vi "FirePneumaticQueue.vi"(8 "error in (no error)":errorcluster, 10 "Variant":variant) -> (0 "error out":errorcluster)   [LabVIEW 2012]
uses:
  RefnameEnum.ctl
  <vilib>/Rock Robotics/WPI/Solenoid/WPI_SolenoidValue.ctl
  <vilib>/Rock Robotics/WPI/Solenoid/WPI_SolenoidSetEnum.vi
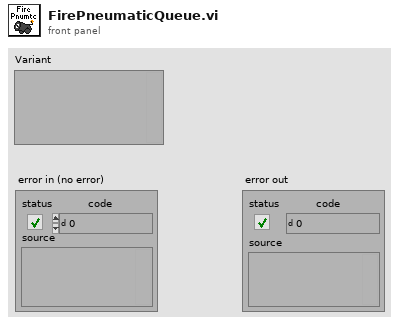
[diagram p1: front panel]
types:
  T1 = typedef "WPI_SolenoidValue.ctl" = enum16{"Off", "On", "Forward", "Reverse"}
  T2 = typedef "RefnameEnum.ctl" = enum16{"FireLauncher", "Climber", "Shield", "TankDrive", "DriveEncoderL", "DriveEncoderR", "LauncherMotorRPM", "LauncherEncoderAnalog", "LauncherEncoderRPM", "ShooterLS", "DriveAlignLSLeft", "DriveAlignLSRight", "ClimbingLS", "LauncherEncoderAngle", "LauncherMotorAngle", "Gamepad1", "Gamepad2", "Compressor", "ClimbWeightSol3", "ClimbWeightSol4"}
  T3 = typedef "WPI_SolenoidDevRef.ctl" = cluster{"DevStatus":errorcluster, "Solenoid Module":T4, "Forward Solenoid Channel":T5, "Reverse Solenoid Channel":T5}
  T4 = typedef "FPGA_TypedefSolenoidModule.ctl" = enum16{"Solenoid Module 1", "Solenoid Module 2"}
  T5 = typedef "WPI_SolenoidChannel.ctl" = enum8{"Solenoid 1", "Solenoid 2", "Solenoid 3", "Solenoid 4", "Solenoid 5", "Solenoid 6", "Solenoid 7", "Solenoid 8", "Invalid"}
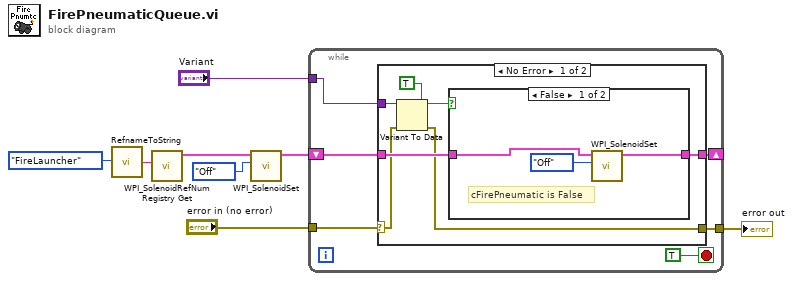
[diagram p0: block diagram]
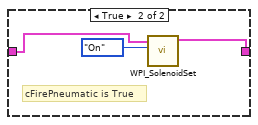
[diagram p2: hidden frame]
diagram:
  n1 = call "RefnameToString.vi"("Enum"=RefnameEnum."FireLauncher") -> ("Refname"=w6:string)
  n2 = call <vilib>:"WPI_SolenoidRefNum Registry Get.vi"("refnum name"=w6) -> ("SolenoidDevRef"=w8:T3)  [unwired: 9 in, 1 out]
  n3 = call-poly <vilib>:"WPI_SolenoidSet.vi"("Value"=WPI_SolenoidValue."Off", "SolenoidDevRef"=w8) -> ("SolenoidDevRef"=w5:T3)  [unwired: 1 in, 8 out]
  n4 = while {
    shift-right: [w13] -> _
    shift-left: w5 -> [w14]
    tunnel: "Variant" -> [w10]
    tunnel: "error in (no error)" -> [w11]
    tunnel: [w9] -> w1
    stop <- TRUE stop-if-true
    n5 = case shown="No Error" w11 {
      selector: w11 -> [w17 w28]
      tunnel: w14 -> [w19 w29]
      tunnel: [w18 w29] -> w13
      tunnel: w10 -> [w16 _]
      tunnel: [w15 w28] -> w9
      frame No Error {
        n6 = Variant To Data(error in=w17, type=TRUE, Variant=w16) -> (data=w20:bool, error out=w15:errorcluster)
        n7 = case shown="False" w20 {
          tunnel: w19 -> [w23 w26]
          tunnel: [w22 w25] -> w18
          frame False {
            # "cFirePneumatic is False"
            n8 = call-poly <vilib>:"WPI_SolenoidSet.vi"("Value"=WPI_SolenoidValue."Off", "SolenoidDevRef"=w23) -> ("SolenoidDevRef"=w22:T3)  [unwired: 1 in, 8 out]
          }
          frame True {
            # "cFirePneumatic is True"
            n9 = call-poly <vilib>:"WPI_SolenoidSet.vi"("Value"=WPI_SolenoidValue."On", "SolenoidDevRef"=w26) -> ("SolenoidDevRef"=w25:T3)  [unwired: 1 in, 8 out]
          }
        }
      }
      frame Error {
      }
    }
  }
  "error out" <- w1
